vi "create.events.vi"(8 "error in (no error)":errorcluster, 11 "EventDaemon in":refnum<class "ErrorHandler.lvclass">) -> (0 "error out":errorcluster, 3 "EventDaemon out":refnum<class "ErrorHandler.lvclass">)   [LabVIEW 2024, in "ErrorHandler.lvclass"]
doc: "Create all event-based messaging."
uses:
  ErrorHandler.lvclass
  ErrorHandler.lvclass/ErrorHandler.ctl
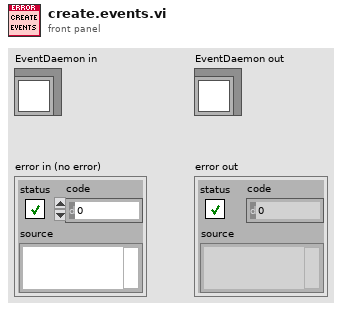
[diagram p1: front panel]
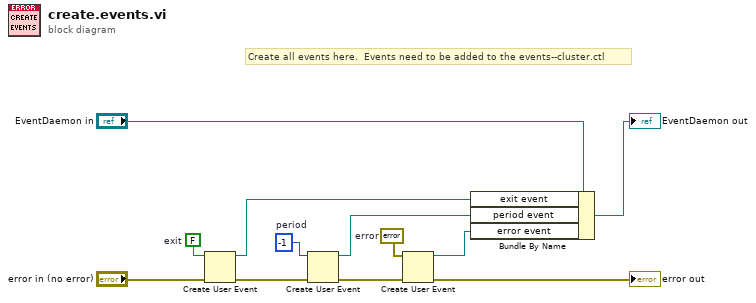
[diagram p0: block diagram]
diagram:
  w4 = errorcluster {"status"=FALSE, "code"=0, "source"=""}  # error
  w7 = -1  # period
  w10 = FALSE  # exit
  # "Create all events here.  Events need to be added to the events--cluster.ctl"
  n1 = Create User Event(user event datatype=w10, error in="error in (no error)") -> (user event=w9:refnum<user-event>, error out=w6:errorcluster)
  n2 = Create User Event(user event datatype=w7, error in=w6) -> (user event=w5:refnum<user-event>, error out=w3:errorcluster)
  n3 = Create User Event(user event datatype=w4, error in=w3) -> (user event=w1:refnum<user-event>, error out=→"error out":errorcluster)
  n4 = Bundle By Name(cluster="EventDaemon in", "exit event"=w9, "period event"=w5, "error event"=w1) -> (→"EventDaemon out":refnum<class "ErrorHandler.lvclass">)
